vi "Create CSI-2 Packet TDMS Files _ looponsettings.vi"() -> ()   [LabVIEW 2025, in "GettingStarted_Gen_148X_Host.lvlib"]
uses:
  GettingStarted_Gen_148X_Host.lvlib
  Types/Frame Data Configuration.ctl
  <instrlib>/FlexRIO/CSI-2/v2/Common/Types/LLP Data Type.ctl
  Types/Frame Timing Configuration.ctl
  Common/GettingStarted_Common_148X_Host.lvlib
  <instrlib>/FlexRIO/CSI-2/v2/Common/NI CSI-2 API Common v2.lvlib
panel:
  out "created path":path
  out "Actrual Frame":i32
  in  "Generate LLP Packet Offsets":bool=TRUE
  in  "Serial Input Channels":string[](array[string])=["SI0"]
  out "Actual Frame Rate (fps)":dbl
  in  "Frame Timing Configuration":T1={"desired frame rate (fps)"=30.0, "actual link data rate (B/s)"=385000000.0, "minimum delay between packets (cycles)"=500, "line blanking (cycles)"=1000} {"actual link data rate (B/s)" format="%_6p"; "line blanking (cycles)" format="%#.0f"}
  in  "Number of Frames":i32=10
  in  "Frame Data Configuration":T2[](array[typedef])=[{"pixel data type"=enum."RAW 8", "horizontal resolution"=1920, "vertical resolution"=1080, "virtual channel"=0.0, "include line sync packets"=FALSE}, {"pixel data type"=enum."RAW 8", "horizontal resolution"=800, "vertical resolution"=600, "virtual channel"=0.0, "include line sync packets"=FALSE}, {"pixel data type"=enum."RAW 8", "horizontal resolution"=3840, "vertical resolution"=2160, "virtual channel"=0.0, "include line sync packets"=FALSE}]
  out "Error Out":errorcluster
  in  "TDMS File Directory":path
  # "Overview: Create sample TDMS files for use with the Generation Getting Started example.  \nInstructions: Visit https://ni.com/r/automotive-camera-module-ref for a detailed tutorial or use the basic instructions below.\n\n 1. Select the serial input channel names to use when creating the files.  The Generation Getting Started example expects the serial input channel number of the file to match the serial output channel number used to generate the data.\n 2. Select the destination directory for the created TDMS files.  Leave blank to use the \"TDMS Files\" directory in the same directory as this VI.\n 3. Select the number of frames to create. \n 4. Select the frame data configuration.  This determines what the frames will look like.  Each frame will be identical with the exception of the frame number.  Each line within a frame will be identical with the exception of the line number (if configured to send line sync packets).  The packet payload is a byte ramp; this is independent of the pixel data type.\n 5. Select the frame timing configuration.  This determines the timing of the individual packets.  The Actual Frame Rate (fps) indicator shows the frame rate of the generated data.  It is possible that this will be lower than the desired frame rate because the interpacket delay cycles and line blanking cycles  are priortized over the frame rate."
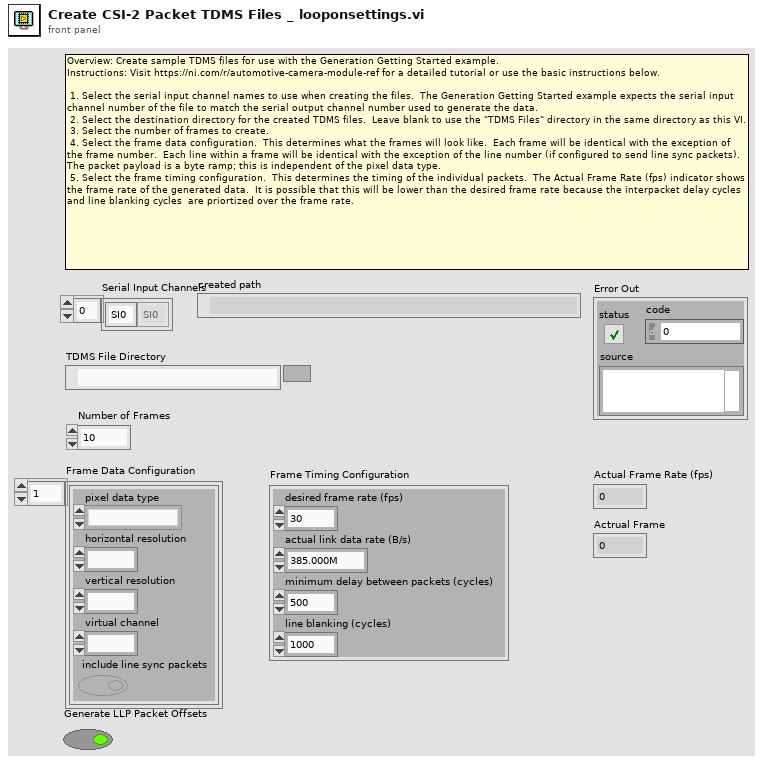
[diagram p1: front panel]
types:
  T1 = typedef "GettingStarted_Gen_148X_Host.lvlib/Frame Timing Configuration.ctl" = cluster{"desired frame rate (fps)":dbl, "actual link data rate (B/s)":dbl, "minimum delay between packets (cycles)":u64, "line blanking (cycles)":u64}
  T2 = typedef "GettingStarted_Gen_148X_Host.lvlib/Frame Data Configuration.ctl" = cluster{"pixel data type":T3, "horizontal resolution":u16, "vertical resolution":u16, "virtual channel":fxp<+,4,4>, "include line sync packets":bool}
  T3 = typedef "NI CSI-2 API Common v2.lvlib/LLP Data Type.ctl" = enum8{"Frame Start", "Frame End", "Line Start", "Line End", "End of Transmission", "Reserved 0", "Reserved 1", "Reserved 2", "Generic Short Packet 1", "Generic Short Packet 2", "Generic Short Packet 3", "Generic Short Packet 4", "Generic Short Packet 5", "Generic Short Packet 6", "Generic Short Packet 7", "Generic Short Packet 8", "Null", "Blanking Data", "Embedded 8-bit non Image Data", "Generic Long Packet 1", "Generic Long Packet 2", "Generic Long Packet 3", "Generic Long Packet 4", "Reserved 3", "YUV420 8-bit", "YUV420 10-bit", "Legacy YUV420 8-bit", "Reserved 4", "YUV420 8-bit Chroma Shifted", "YUV420 10-bit Chroma Shifted", "YUV422 8-bit", "YUV422 10-bit", "RGB444", "RGB555", "RGB565", "RGB666", "RGB888", "Reserved 5", "Reserved 6", "RAW 24", "RAW 6", "RAW 7", "RAW 8", "RAW 10", "RAW 12", "RAW 14", "RAW 16", "RAW 20", "User Defined 8-bit Data 1", "User Defined 8-bit Data 2", "User Defined 8-bit Data 3", "User Defined 8-bit Data 4", "User Defined 8-bit Data 5", "User Defined 8-bit Data 6", "User Defined 8-bit Data 7", "User Defined 8-bit Data 8", "USL Command", "Reserved 7", "Reserved 8", "Reserved 9", "Reserved 10", "Reserved 11", "Reserved 12", "LRTE EPD Spacer"}
  T4 = enum16{"open", "open or create", "create or replace", "create", "open (read-only)"}
  T5 = enum16{"big-endian, network order", "native, host order", "little-endian"}
  T6 = typedef "NI CSI-2 API Host v2.lvlib/Host LLP Packet.ctl" = cluster{"header":T7, "payload":u8[], "footer":T8}
  T7 = typedef "NI CSI-2 API FPGA v2.lvlib/LLP Packet Header.ctl" = cluster{"word count":u16, "ecc":fxp<+,6,6>, "vcx":fxp<+,2,2>, "data type":fxp<+,6,6>, "vc":fxp<+,2,2>}
  T8 = typedef "NI CSI-2 API FPGA v2.lvlib/LLP Packet Footer.ctl" = cluster{"crc":u16}
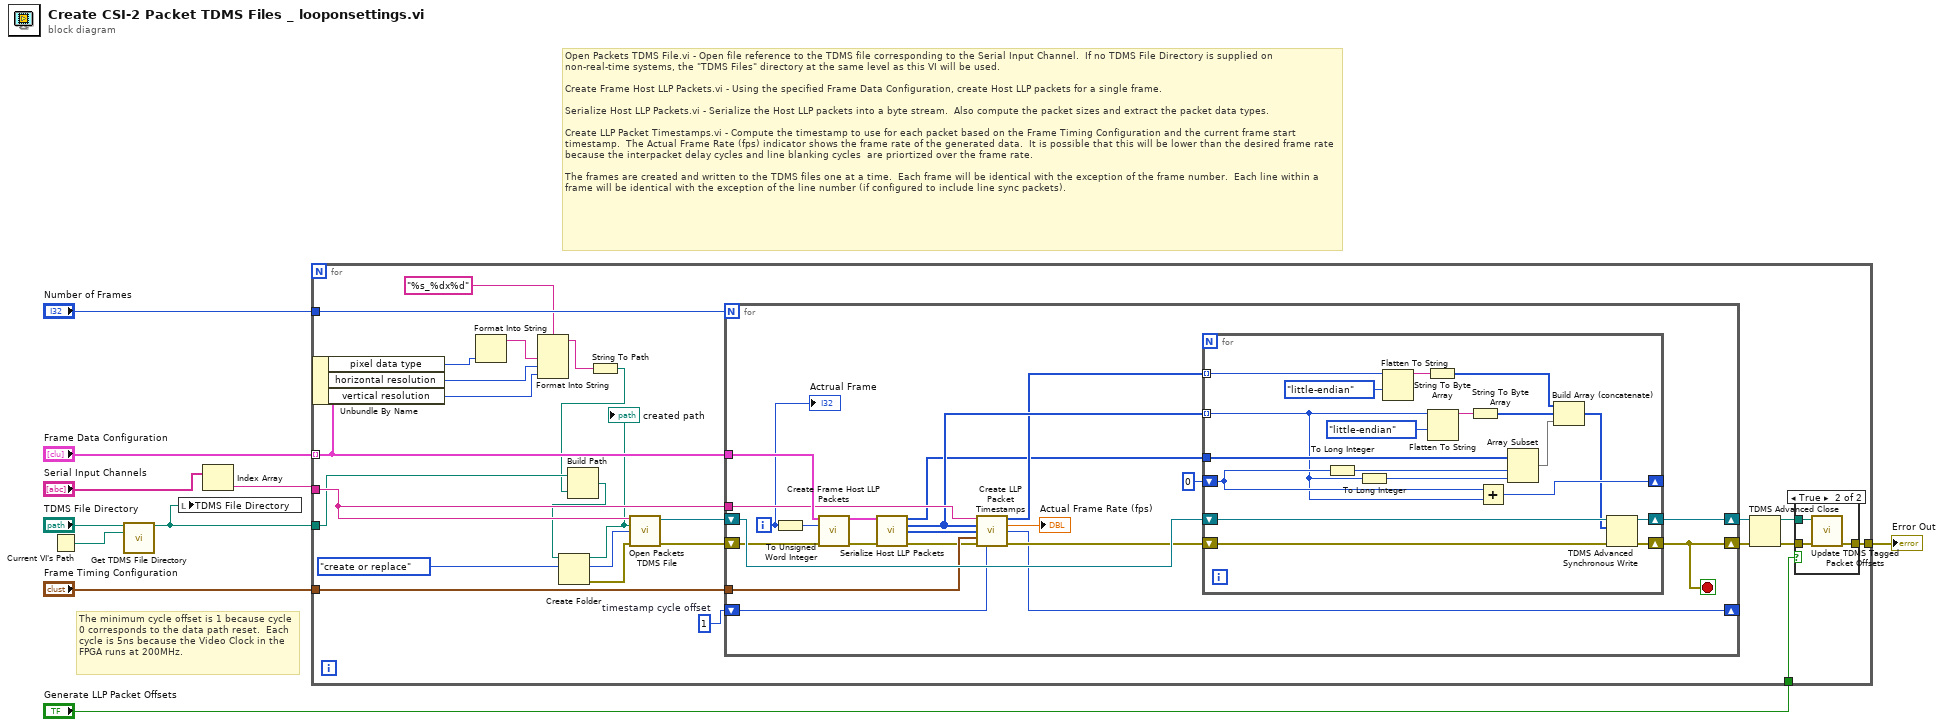
[diagram p0: block diagram]
diagram:
  # "The minimum cycle offset is 1 because cycle 0 corresponds to the data path reset.  Each cycle is 5ns because the Video Clock in the FPGA runs at 200MHz."
  # "Open Packets TDMS File.vi - Open file reference to the TDMS file corresponding to the Serial Input Channel.  If no TDMS File Directory is supplied on non-real-time systems, the \"TDMS Files\" directory at the same level as this VI will be used.\n\nCreate Frame Host LLP Packets.vi - Using the specified Frame Data Configuration, create Host LLP packets for a single frame.\n\nSerialize Host LLP Packets.vi - Serialize the Host LLP packets into a byte stream.  Also compute the packet sizes and extract the packet data types. \n\nCreate LLP Packet Timestamps.vi - Compute the timestamp to use for each packet based on the Frame Timing Configuration and the current frame start timestamp.  The Actual Frame Rate (fps) indicator shows the frame rate of the generated data.  It is possible that this will be lower than the desired frame rate because the interpacket delay cycles and line blanking cycles  are priortized over the frame rate.\n\nThe frames are created and written to the TDMS files one at a time.  Each frame will be identical with the exception of the frame number.  Each line within a frame will be identical with the exception of the line number (if configured to include line sync packets)."
  n1 = Current VI's Path() -> (path=w5:path)
  n2 = call "Get TDMS File Directory.vi"("tdms file directory in"="TDMS File Directory", "calling vi path"=w5) -> ("tdms file directory out"=w7:path)  [unwired: 13 in]
  n3 = local write "TDMS File Directory"(w7) -> ()
  n4 = Index Array(array="Serial Input Channels") -> (element=w1:string)  [unwired: 1 in]
  n5 = for {
    tunnel: [w24] -> w4
    tunnel: "Frame Data Configuration" -> [w22] mode=indexing
    tunnel: "Number of Frames" -> [w35]
    tunnel: "Frame Timing Configuration" -> [w34]
    tunnel: w7 -> [w14]
    tunnel: w1 -> [w30]
    tunnel: "Generate LLP Packet Offsets" -> [w23]
    w31 = u64 1  # timestamp cycle offset
    n6 = Unbundle By Name(w22) -> ("pixel data type"=w20:T3, "horizontal resolution"=w18:u16, "vertical resolution"=w17:u16)
    n7 = Format Into String(w20) -> (resulting string=w19:string)  [unwired: 3 in, 1 out]
    n8 = Format Into String(format string="%s_%dx%d", w19, w18, w17) -> (resulting string=w13:string)  [unwired: 2 in, 1 out]
    n9 = String To Path(string=w13) -> (path=w12:path)
    n10 = Build Path(base path=w14, name or relative path=w12) -> (appended path=w11:path)
    n11 = Create Folder(path (use dialog)=w11) -> (created path=w15:path, error out=w16:errorcluster)  [unwired: 2 in, 1 out]
    "created path" <- w15
    n12 = call "Open Packets TDMS File.vi"("serial input channel"=w30, "base tdms file path"=w15, "file operation type"=T4."create or replace", "error in"=w16) -> ("packets file ref"=w32:refnum<k34>, "error out"=w29:errorcluster)  [unwired: 10 in]
    n13 = for {
      N: w35 -> [_]
      tunnel: w22 -> [w59]
      tunnel: w30 -> [w57]
      shift-right: [w44] -> w33
      shift-left: w32 -> [w60]
      shift-right: [w54] -> _
      shift-left: w31 -> [w52]
      tunnel: w34 -> [w51]
      shift-right: [w45] -> w27
      shift-left: w29 -> [w58]
      i -> [w40]
      stop <- w45 stop-if-true
      n14 = To Unsigned Word Integer(number=w40) -> (unsigned 16bit integer=w55:u16)
      n15 = call "Create Frame Host LLP Packets.vi"("frame configuration"=w59, "frame number"=w55, "error in (no error)"=w58) -> ("frame packets"=w50:T6[], "error out"=w49:errorcluster)  [unwired: 11 in]
      n16 = call "Serialize Host LLP Packets.vi"("host llp packets"=w50, "error in (no error)"=w49) -> ("packet bytes"=w42:u8[], "packet sizes"=w48:u32[], "packet data types"=w47:T3[], "error out"=w46:errorcluster)  [unwired: 10 in]
      n17 = call "Create LLP Packet Timestamps.vi"("serial input channel"=w57, "llp packet sizes"=w48, "packet data types"=w47, "frame timing configuration"=w51, "error in (no error)"=w46, "frame start timestamp"=w52) -> ("timestamps"=w43:u64[], "actual frame rate (fps)"=→"Actual Frame Rate (fps)":dbl, "next frame start timestamp"=w54:u64, "error out"=w56:errorcluster)  [unwired: 6 in]
      n18 = for {
        tunnel: w48 -> [w69] mode=indexing
        tunnel: w43 -> [w79] mode=indexing
        shift-right: [w63] -> w44
        shift-left: w60 -> [w64]
        shift-right: [w65] -> w45
        shift-left: w56 -> [w62]
        shift-right: [w76] -> _
        shift-left: u32 0 -> [w74]
        tunnel: w42 -> [w75]
        n19 = To Long Integer(number=w74) -> (32bit integer=w71:i32)
        n20 = To Long Integer(number=w69) -> (32bit integer=w70:i32)
        n21 = Flatten To String(anything=w79, byte order (0:big-endian, network order)=T5."little-endian") -> (data string=w78:string)  [unwired: 2 in, 2 out]
        n22 = String To Byte Array(string=w78) -> (unsigned byte array=w66:u8[])
        n23 = Flatten To String(anything=w69, byte order (0:big-endian, network order)=T5."little-endian") -> (data string=w77:string)  [unwired: 2 in, 2 out]
        n24 = String To Byte Array(string=w77) -> (unsigned byte array=w67:u8[])
        n25 = Add(x=w74, y=w69) -> (x+y=w76:u32)
        n26 = Array Subset(array=w75, index=w71, length=w70) -> (w68:u8[])
        n27 = Build Array (concatenate)(w66, w67, w68) -> (w61:u8[])
        n28 = TDMS Advanced Synchronous Write(8:w62, 10:w61, 11:w64) -> (0:w65:errorcluster, 3:w63:refnum<k34>)
      }
      "Actrual Frame" <- w40
    }
    n29 = TDMS Advanced Close(8:w27, 11:w33) -> (0:w25:errorcluster, 3:w26:path)  [unwired: 2 in]
    n30 = case shown="True" w23 {
      tunnel: w26 -> [_ w39]
      tunnel: w25 -> [w36 w38]
      tunnel: [w36 w37] -> w24
      frame False {
      }
      frame True {
        n31 = call "Update TDMS Tagged Packet Offsets.vi"("llp tagged packet file path"=w39, "error in"=w38) -> ("error out"=w37:errorcluster)  [unwired: 12 in, 1 out]
      }
    }
  }
  "Error Out" <- w4
